vi "live view D05.vi"() -> ()   [LabVIEW 2019, in "D05.lvlib"]
uses:
  D05.lvlib
  <vilib>/userDefined/High Color/IMAQdx.ctl
  <vilib>/vision/Image Controls.llb/IMAQ Image.ctl
  <vilib>/measure/mamon.llb/Trigger Detection for 1 Channel.vi
  <vilib>/measure/NI_MAPro.lvlib
  Calibration Lib.lvlib
  database.lvlib
  <vilib>/vision/driver/NI_Vision_Acquisition_Software.lvlib
panel:
  out "error out":errorcluster
  in  "snapshot":bool
  out "projector D30 error":errorcluster
  in  "Path":path
  in  "Verify Calibration D29":bool caption="capture grab"
  out "factor":sgl
  out "transform matrix":sgl[](array[numeric])
  in  "Method 2 save D30":bool caption="capture grab"
  in  "Method 1 Save D30":bool caption="Saving txt"
  in  "Close":bool
  out "Average Result":string="Average Result"
  out ">18  A":dbl(slide)=1.0 caption=">18 mm" scale=0.0..100.0
  out "16-18  A":dbl(slide)=1.0 caption="16-18 mm" scale=0.0..100.0
  out "14-16  A":dbl(slide)=1.0 caption="14-16 mm" scale=0.0..100.0
  out "12.5-14 A":dbl(slide)=1.0 caption="12.5-14 mm" scale=0.0..100.0
  out "10-12.5  A":dbl(slide)=1.0 caption="10-12.5 mm" scale=0.0..100.0 scale format="%#_4f"
  out "8-10  A":dbl(slide)=1.0 caption="8-10 mm" scale=0.0..100.0
  out "6.3-8  A":dbl(slide)=1.0 caption="6.3-8 mm" scale=0.0..100.0
  out "<6.3  A":dbl(slide)=1.0 caption="<6.3 mm" scale=0.0..100.0
  out "Live Result":string="Live Result"
  out ">18  L":dbl(slide)=1.0 caption=">18 mm" scale=0.0..100.0
  out "Live View":T1(plugin-control) caption="Disc 26"
  out "16-18  L":dbl(slide)=1.0 caption="16-18 mm" scale=0.0..100.0
  out "14-16  L":dbl(slide)=1.0 caption="14-16 mm" scale=0.0..100.0
  out "12.5-14 L":dbl(slide)=1.0 caption="12.5-14 mm" scale=0.0..100.0
  out "10-12.5  L":dbl(slide)=1.0 caption="10-12.5 mm" scale=0.0..100.0 scale format="%#_4f"
  out "8-10  L":dbl(slide)=1.0 caption="8-10 mm" scale=0.0..100.0
  out "6.3-8  L":dbl(slide)=1.0 caption="6.3-8 mm" scale=0.0..100.0
  out "<6.3  L":dbl(slide)=1.0 caption="<6.3 mm" scale=0.0..100.0
  out "disc name":string="Live Info Disc 05"
  out "dsgs":string="DSGS"
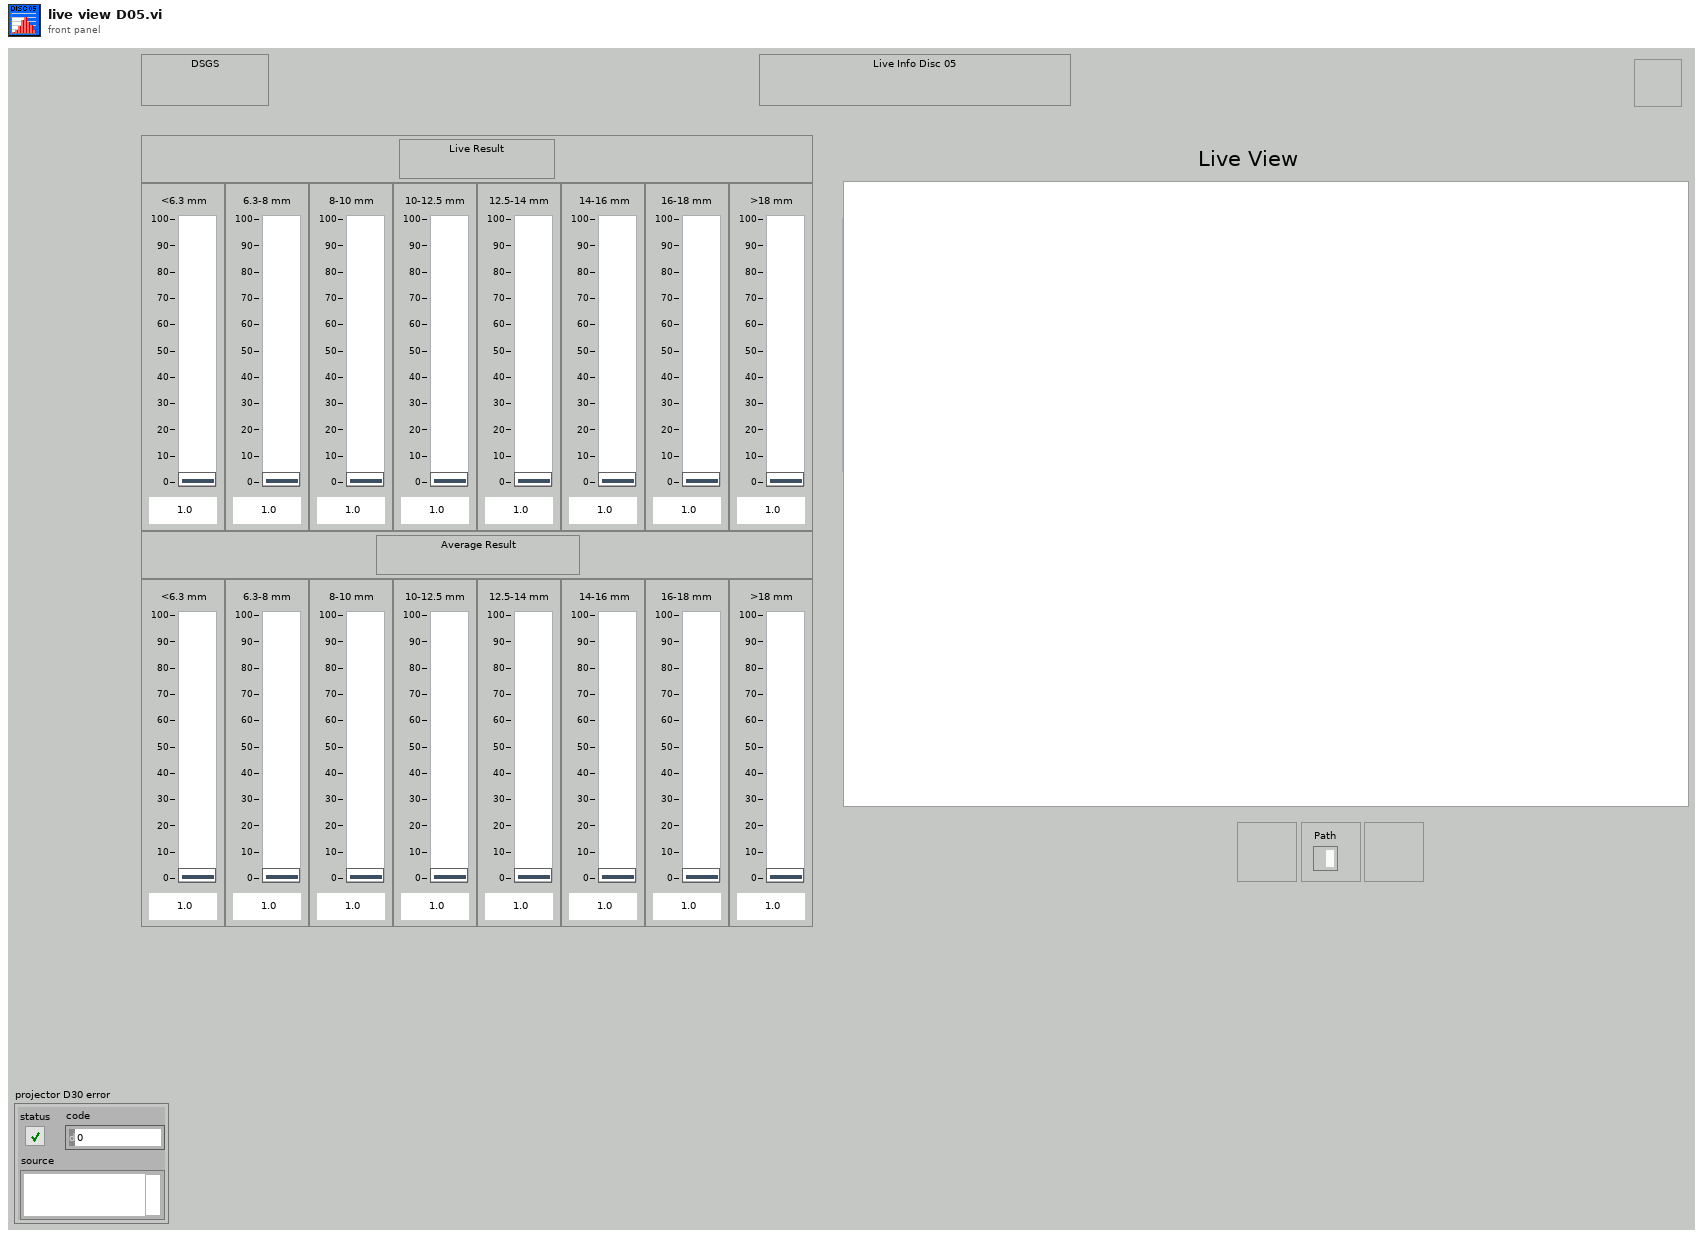
[diagram p1: front panel]
types:
  T1 = typedef "IMAQ Image.ctl" = refnum<image>
  T2 = typedef "IMAQdx.ctl" = refnum<k21>
  T3 = enum8{"Enabled", "Disabled", "Disabled and Grayed Out"}
  T4 = cluster{"date/time string":string, "date/time string":string, "date/time string":string, string, "spreadsheet string":string, string}
  T5 = cluster{"date/time string":string, "date/time string":string, string, "Value":dbl, "Value":dbl, "Value":dbl, "Value":dbl, "Value":dbl, "Value":dbl, "Value":dbl, "Value":dbl}
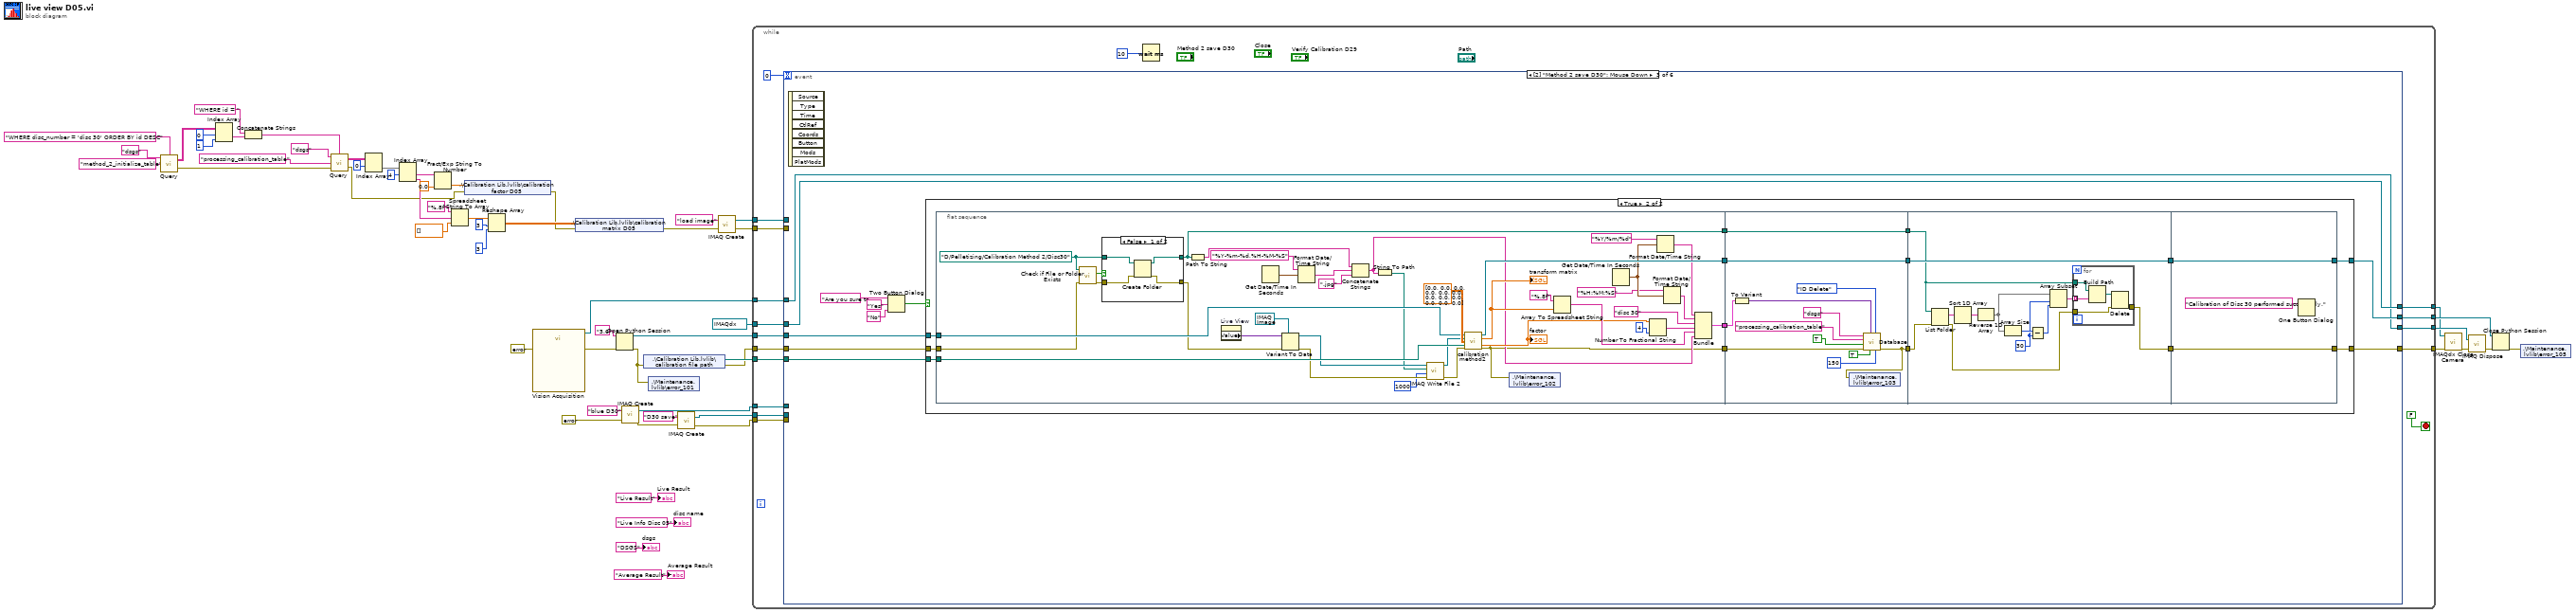
[diagram p0: block diagram]
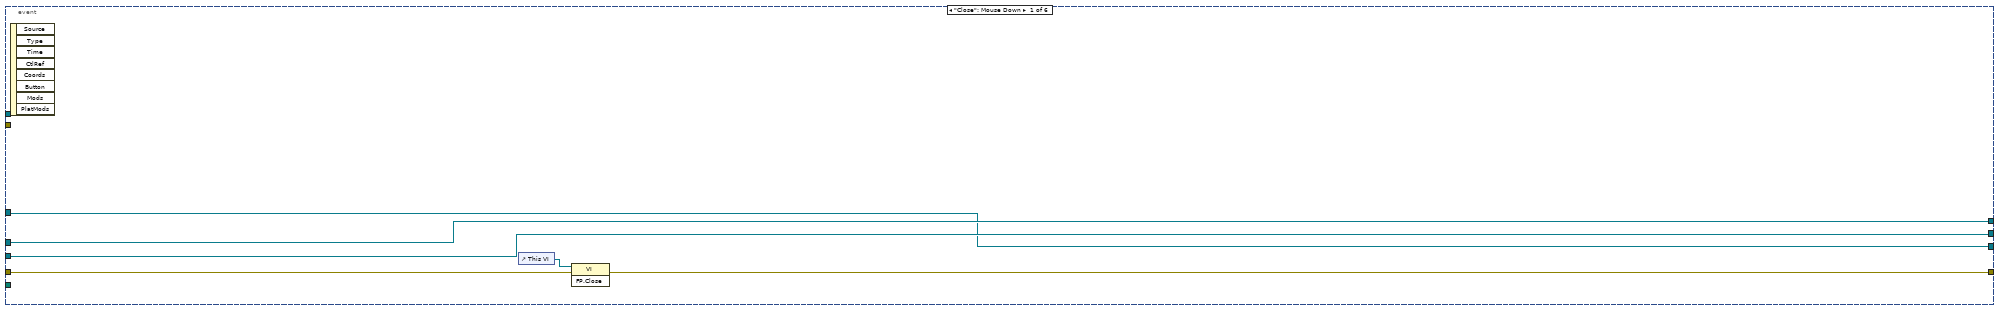
[diagram p2: hidden frame]
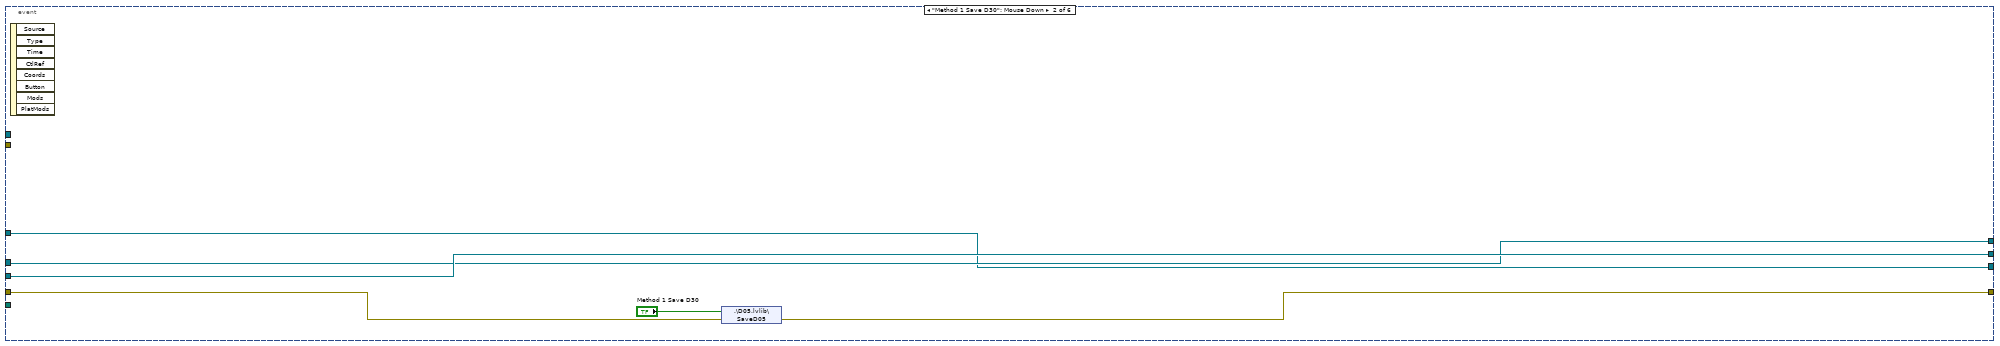
[diagram p3: hidden frame]
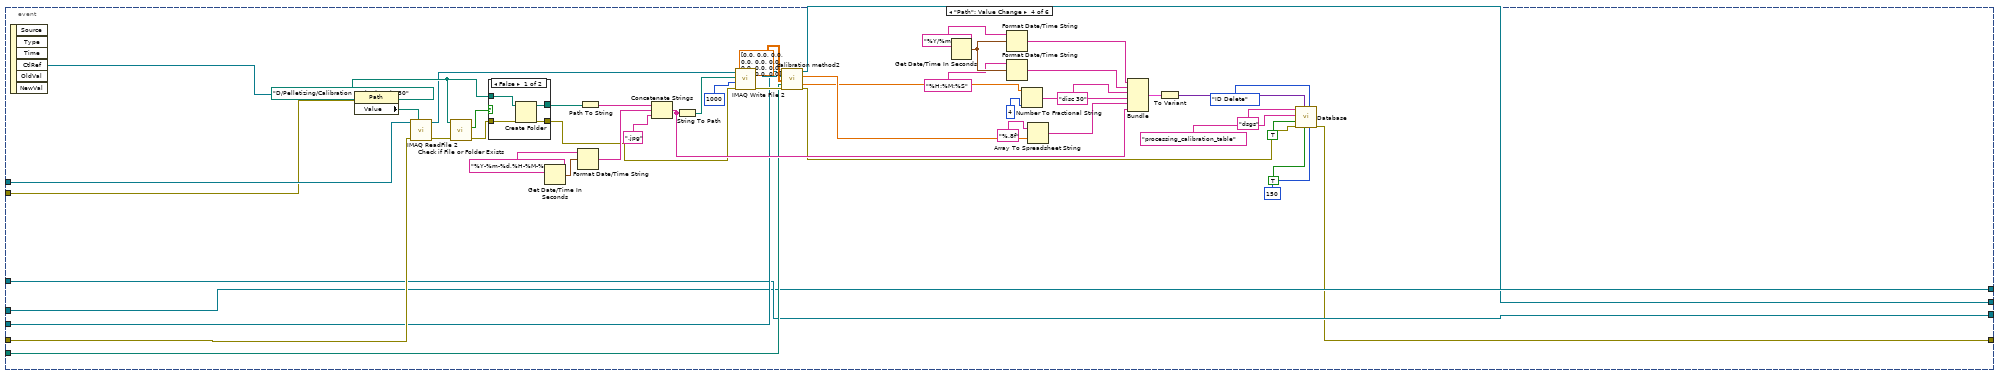
[diagram p6: hidden frame]
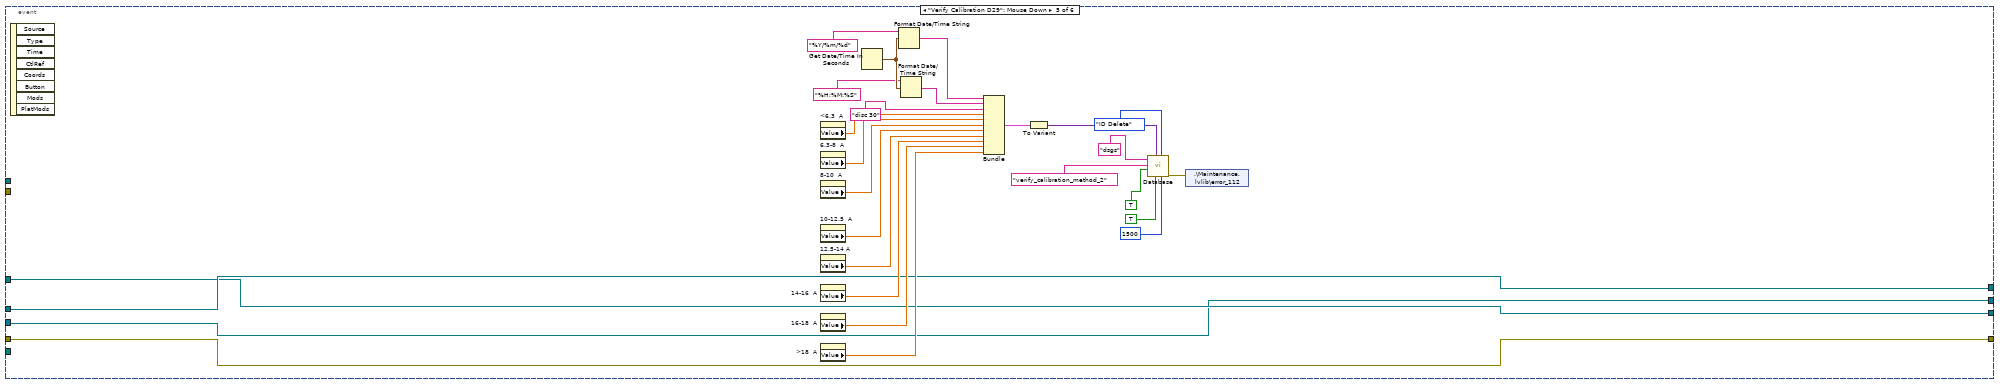
[diagram p8: hidden frame]
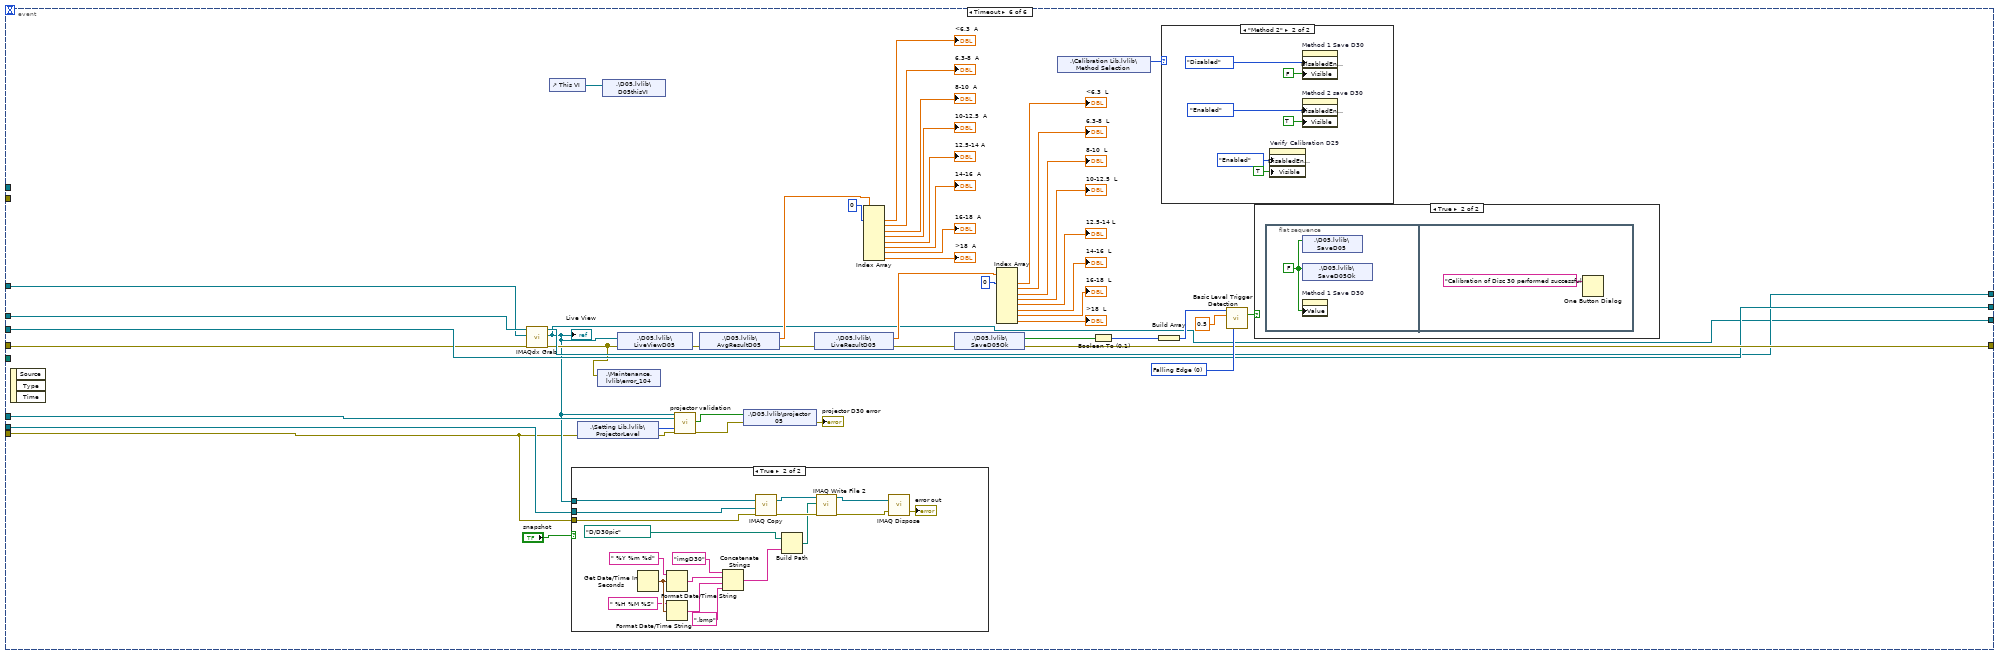
[diagram p9: hidden frame]
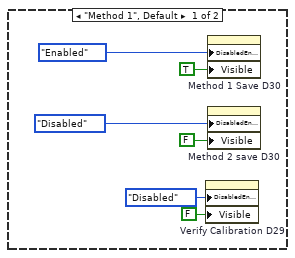
[diagram p11: hidden frame]
diagram:
  n1 = call "Query.vi"("Condition"="WHERE disc_number = 'disc 30' ORDER BY id DESC", "Table Name"="method_2_initialize_table", "Connection Name"="dsgs") -> ("Error out"=w28:errorcluster, "data"=w33:string[][])  [unwired: 1 in]
  n2 = Index Array(array=w33, index (row)=0, index (col)=1 ("disabled index (col)")) -> (element=w26:string)
  n3 = Concatenate Strings("WHERE id = " ("string"), w26) -> (w25:string)
  n4 = call "Query.vi"("Condition"=w25, "Error in"=w28, "Table Name"="processing_calibration_table", "Connection Name"="dsgs") -> ("Error out"=w9:errorcluster, "data"=w24:string[][])
  n5 = Index Array(array=w24, index (row)=0) -> (element=w22:string[])  [unwired: 1 in]
  n6 = Index Array(array=w22, index #1=4 ("index")) -> (element #1=w20:string, element #2=w12:string)  [unwired: 1 in]
  n7 = Fract/Exp String To Number(string=w20, default (0 dbl)=sgl 0.0 ("default (0 DBL)")) -> (number=w19:sgl)  [unwired: 2 in, 1 out]
  n8 = Spreadsheet String To Array(format string="%.8f", spreadsheet string=w12, array type (2D Dbl)=sgl[] []) -> (array=w16:sgl[])  [unwired: 1 in]
  n9 = shared-variable ".\\Calibration Lib.lvlib\\calibration factor D05"(w19, error in=w9) -> (error out=w10:errorcluster)
  n10 = Reshape Array(w16, 3 ("dimension size"), 3 ("dimension size")) -> (w11:sgl[][])
  n11 = call "Vision Acquisition"("error in"=errorcluster {"status"=FALSE, "code"=0, "source"=""}) -> ("Image Out"=w45:T1, "error out"=w44:errorcluster)  [unwired: 24 in, 1 out]
  n12 = shared-variable ".\\Calibration Lib.lvlib\\calibration matrix D05"(w11, error in=w10) -> (error out=w8:errorcluster)
  n13 = Open Python Session(python version="3.6" ("Python version"), 3:w44) -> (session out=w54:refnum<k35>, error out=w40:errorcluster)  [unwired: 1 in]
  n14 = call "IMAQ Create"("Image Name"="blue D30", "error in (no error)"=errorcluster {"status"=FALSE, "code"=0, "source"=""}) -> ("New Image"=w5:T1, "error out"=w4:errorcluster)  [unwired: 3 in]
  n15 = shared-variable ".\\Calibration Lib.lvlib\\calibration file path"(error in=w40) -> (w43:path, error out=w42:errorcluster)
  n16 = shared-variable ".\\Maintenance.lvlib\\error_101"(w40) -> ()  [unwired: 1 in, 1 out]
  n17 = call "IMAQ Create"("Image Name"="D30 save", "error in (no error)"=w4) -> ("New Image"=w1:T1, "error out"=w3:errorcluster)  [unwired: 3 in]
  n18 = call "IMAQ Create"("Image Name"="load image", "error in (no error)"=w8) -> ("New Image"=w39:T1, "error out"=w38:errorcluster)  [unwired: 3 in]
  n19 = while {
    tunnel: w54 -> [w74]
    tunnel: w43 -> [w73]
    tunnel: w42 -> [w72]
    tunnel: w45 -> [w70]
    tunnel: [w69] -> w53
    tunnel: [w68] -> w50
    tunnel: [w67] -> w52
    tunnel: T2 "disc30" ("Session In") -> [w66]
    tunnel: [w65] -> w47
    tunnel: w39 -> [w64]
    tunnel: w38 -> [w63]
    tunnel: w5 -> [w62]
    tunnel: w3 -> [w61]
    tunnel: w1 -> [w60]
    stop <- FALSE stop-if-true
    n20 = event shown="[2] \"Method 2 save D30\": Mouse Down" {
      selector: _ -> [_ _ _ _ _ _]
      dyn-events: _ -> [_ _ _ _ _ _]
      timeout: 0 -> [_ _ _ _ _ _]
      tunnel: w74 -> [w80 w86 w99 w196 w250 w290]
      tunnel: w73 -> [_ _ w98 w197 _ _]
      tunnel: [w82 w88 w93 w193 w253 w293] -> w68
      tunnel: w72 -> [w81 w87 w97 w198 w253 w286]
      tunnel: w70 -> [w77 w84 w94 w195 w251 w288]
      tunnel: [w77 w84 w94 w195 w251 w277] -> w69
      tunnel: [w80 w86 w96 w192 w250 w290] -> w67
      tunnel: w66 -> [w78 w85 w95 w194 w252 w289]
      tunnel: [w78 w85 w95 w194 w252 w287] -> w65
      tunnel: w64 -> [_ _ _ w200 _ _]
      tunnel: w63 -> [_ _ _ w199 _ _]
      tunnel: w62 -> [_ _ _ _ _ w279]
      tunnel: w61 -> [_ _ _ _ _ w275]
      tunnel: w60 -> [_ _ _ _ _ w276]
      event "Close": Mouse Down {
        n21 = event-data() -> ()  [unwired: 1 in, 8 out]
        n22 = control-ref of="This VI"() -> (w79:refnum<vi>)
        n23 = invoke class="VI" method="FP.Close"(reference=w79, error in=w81) -> (error out=w82:errorcluster)  [unwired: 1 in, 2 out]
      }
      event "Method 1 Save D30": Mouse Down {
        n24 = event-data() -> ()  [unwired: 1 in, 8 out]
        n25 = shared-variable ".\\D05.lvlib\\SaveD05"("Method 1 Save D30", error in=w87) -> (error out=w88:errorcluster)
      }
      event "Method 2 save D30": Mouse Down {
        n26 = event-data() -> ()  [unwired: 1 in, 8 out]
        n27 = Two Button Dialog(message="Are you sure to calibration Disc 30?", 1:"No" ("F button name (\"Cancel\")"), 2:"Yes" ("T button name (\"OK\")")) -> (T button?=w89:bool)
        n28 = case shown="True" w89 {
          tunnel: w99 -> [w100 w108]
          tunnel: w98 -> [_ w107]
          tunnel: w97 -> [w101 w106]
          tunnel: [w100 w105] -> w96
          tunnel: [w101 w104] -> w93
          frame False {
          }
          frame True {
            n29 = flat-sequence {
              tunnel: [w153] -> w115
              tunnel: [w119] -> w114
              tunnel: [w144] -> w113
              tunnel: w106 -> [w125]
              tunnel: w107 -> [w143]
              tunnel: w108 -> [w135]
              tunnel: [w118] -> w112
              tunnel: w115 -> [w171]
              tunnel: w114 -> [w169]
              tunnel: w113 -> [w164]
              tunnel: [w171] -> w111
              tunnel: [w165] -> w110
              tunnel: [w162] -> w109
              tunnel: w112 -> [w162]
              tunnel: w111 -> [w183]
              tunnel: w110 -> [w173]
              tunnel: w109 -> [w172]
              tunnel: [w183] -> w103
              tunnel: [w174] -> w102
              tunnel: [w190] -> w104
              tunnel: [w191] -> w105
              tunnel: w103 -> [w191]
              tunnel: w102 -> [w190]
              frame #0 {
                w129 = path "D:/Pelletizing/Calibration Method 2/Disc30" ("path")
                n30 = call <vilib>:"Check if File or Folder Exists.vi"("error in (no error)"=w125, "path"=w129) -> ("error out"=w127:errorcluster, "file or folder exists?"=w130:bool)  [unwired: 7 in, 1 out]
                n31 = case shown="False" w130 {
                  tunnel: [w155 w159] -> w118
                  tunnel: w129 -> [w157 w159]
                  tunnel: w127 -> [w156 w158]
                  tunnel: [w154 w158] -> w124
                  frame False {
                    n32 = Create Folder(path (use dialog)=w157, error in=w156) -> (created path=w155:path, error out=w154:errorcluster)  [unwired: 1 in, 1 out]
                  }
                  frame True {
                  }
                }
                n33 = Path To String(path=w118) -> (string=w128:string)
                n34 = property on="Live View" class="ImageControl"() -> ("Value"=w142:variant)  [unwired: 2 in, 2 out]
                n35 = Get Date/Time In Seconds() -> (seconds since 1Jan1904=w134:timestamp)
                n36 = Variant To Data(error in=w124, type=T1 refnum ("New Image"), Variant=w142) -> (data=w123:T1, error out=w122:errorcluster)
                n37 = Format Date/Time String(time format string (%c)="%Y-%m-%d,%H-%M-%S", seconds (now)=w134) -> (date/time string=w132:string)  [unwired: 1 in]
                n38 = Concatenate Strings(w128, w132, ".jpg" ("string")) -> (w126:string)
                n39 = String To Path(string=w126) -> (path=w121:path)
                n40 = call-poly "IMAQ Write File 2"("error in (no error)"=w122, "Image Quality"=u32 1000, "File Path"=w121, "Image"=w123) -> ("error out"=w116:errorcluster, "Image Out (duplicate)"=w117:T1)  [unwired: 6 in]
                n41 = call "calibration method2.vi"("session in"=w135, "Image IN"=w117, "initialize matrix"=sgl[][] [[0.0, 0.0, 0.0], [0.0, 0.0, 0.0], [0.0, 0.0, 0.0], [0.0, 0.0, 0.0]] ("(4*3) array"), "module path"=w143, "error in"=w116) -> ("session out"=w153:refnum<k35>, "calibration vector"=w137:sgl[], "factor"=w139:sgl, "error out"=w119:errorcluster)  [unwired: 6 in, 1 out]
                "factor" <- w139
                "transform matrix" <- w137
                n42 = shared-variable ".\\Maintenance.lvlib\\error_102"(w119) -> ()  [unwired: 1 in, 1 out]
                n43 = Array To Spreadsheet String(array=w137, 3:"%.8f" ("format string")) -> (spreadsheet string=w145:string)  [unwired: 1 in]
                n44 = Get Date/Time In Seconds() -> (seconds since 1Jan1904=w150:timestamp)
                n45 = Number To Fractional String(number=w139, precision (6)=i16 4) -> (F-format string=w146:string)  [unwired: 2 in]
                n46 = Format Date/Time String(time format string (%c)="%Y/%m/%d", seconds (now)=w150) -> (date/time string=w151:string)  [unwired: 1 in]
                n47 = Format Date/Time String(time format string (%c)="%H:%M:%S", seconds (now)=w150) -> (date/time string=w152:string)  [unwired: 1 in]
                n48 = Bundle("date/time string"=w151, "date/time string"=w152, "date/time string"="disc 30", w146, "spreadsheet string"=w145, w126) -> (w144:T4)  [unwired: 1 in]
              }
              frame #1 {
                n49 = To Variant(anything=w164) -> (Variant=w163:variant)
                n50 = call "Database.vi"("Maximum Row"=150, "Enum"=enum16{"ID Delete", "Time Delete"}."ID Delete", "Delete row?"=TRUE, "Data"=w163, "Error in"=w169, "Auto Increment ID?"=TRUE, "Table"="processing_calibration_table", "Connection"="dsgs") -> ("Error out"=w165:errorcluster)  [unwired: 3 in]
                n51 = shared-variable ".\\Maintenance.lvlib\\error_103"(w165) -> ()  [unwired: 1 in, 1 out]
              }
              frame #2 {
                w176 = 30 ("index")
                n52 = List Folder(path=w172, error in=w173) -> (filenames=w177:string[], error out=w175:errorcluster)  [unwired: 2 in, 2 out]
                n53 = Sort 1D Array(array=w177) -> (sorted array=w178:string[])
                n54 = Reverse 1D Array(array=w178) -> (reversed array=w179:string[])
                n55 = Array Size(array=w179) -> (size(s)=w180:i32)
                n56 = Subtract(x=w180, y=w176) -> (x-y=w181:i32)
                n57 = Array Subset(array=w179, index=w176, length=w181) -> (w182:string[])
                n58 = for {
                  tunnel: w182 -> [w187] mode=indexing
                  tunnel: w172 -> [w188]
                  tunnel: [w185] -> w174
                  tunnel: w175 -> [w184]
                  n59 = Build Path(base path=w188, name or relative path=w187) -> (appended path=w186:path)
                  n60 = Delete(path (use dialog)=w186, error in=w184) -> (error out=w185:errorcluster)  [unwired: 3 in, 2 out]
                }
              }
              frame #3 {
                n61 = One Button Dialog(message="Calibration of Disc 30 performed successfully.") -> ()  [unwired: 1 in, 1 out]
              }
            }
          }
        }
      }
      event "Path": Value Change {
        w233 = path "D:/Pelletizing/Calibration Method 2/Disc30" ("path")
        n62 = event-data() -> ("CtlRef"=w201:refnum<vi>)  [unwired: 1 in, 5 out]
        n63 = property class="Path"(reference=w201, error in=w199) -> ("Value"=w228:path)  [unwired: 2 out]
        n64 = call "IMAQ ReadFile 2"("File Path"=w228, "error in (no error)"=w198, "Image"=w200) -> ("error out"=w226:errorcluster, "Image Out"=w227:T1)  [unwired: 4 in, 3 out]
        n65 = call <vilib>:"Check if File or Folder Exists.vi"("error in (no error)"=w226, "path"=w233) -> ("error out"=w230:errorcluster, "file or folder exists?"=w234:bool)  [unwired: 7 in, 1 out]
        n66 = case shown="False" w234 {
          tunnel: [w243 w247] -> w232
          tunnel: w233 -> [w245 w247]
          tunnel: w230 -> [w244 w246]
          tunnel: [w242 w246] -> w203
          frame False {
            n67 = Create Folder(path (use dialog)=w245, error in=w244) -> (created path=w243:path, error out=w242:errorcluster)  [unwired: 1 in, 1 out]
          }
          frame True {
          }
        }
        n68 = Get Date/Time In Seconds() -> (seconds since 1Jan1904=w238:timestamp)
        n69 = Format Date/Time String(time format string (%c)="%Y-%m-%d,%H-%M-%S", seconds (now)=w238) -> (date/time string=w236:string)  [unwired: 1 in]
        n70 = Path To String(path=w232) -> (string=w231:string)
        n71 = Concatenate Strings(w231, w236, ".jpg" ("string")) -> (w214:string)
        n72 = String To Path(string=w214) -> (path=w229:path)
        n73 = call-poly "IMAQ Write File 2"("error in (no error)"=w203, "Image Quality"=u32 1000, "File Path"=w229, "Image"=w227) -> ("error out"=w240:errorcluster, "Image Out (duplicate)"=w225:T1)  [unwired: 6 in]
        n74 = call "calibration method2.vi"("session in"=w196, "Image IN"=w225, "initialize matrix"=sgl[][] [[0.0, 0.0, 0.0], [0.0, 0.0, 0.0], [0.0, 0.0, 0.0], [0.0, 0.0, 0.0]] ("(4*3) array"), "module path"=w197, "error in"=w240) -> ("session out"=w192:refnum<k35>, "calibration vector"=w213:sgl[], "factor"=w212:sgl, "error out"=w202:errorcluster)  [unwired: 6 in, 1 out]
        n75 = Get Date/Time In Seconds() -> (seconds since 1Jan1904=w222:timestamp)
        n76 = Format Date/Time String(time format string (%c)="%Y/%m/%d", seconds (now)=w222) -> (date/time string=w223:string)  [unwired: 1 in]
        n77 = Format Date/Time String(time format string (%c)="%H:%M:%S", seconds (now)=w222) -> (date/time string=w224:string)  [unwired: 1 in]
        n78 = Number To Fractional String(number=w212, precision (6)=i16 4) -> (F-format string=w218:string)  [unwired: 2 in]
        n79 = Array To Spreadsheet String(array=w213, 3:"%.8f" ("format string")) -> (spreadsheet string=w217:string)  [unwired: 1 in]
        n80 = Bundle("date/time string"=w223, "date/time string"=w224, "date/time string"="disc 30", w218, "spreadsheet string"=w217, w214) -> (w204:T4)  [unwired: 1 in]
        n81 = To Variant(anything=w204) -> (Variant=w207:variant)
        n82 = call "Database.vi"("Maximum Row"=150, "Enum"=enum16{"ID Delete", "Time Delete"}."ID Delete", "Delete row?"=TRUE, "Data"=w207, "Error in"=w202, "Auto Increment ID?"=TRUE, "Table"="processing_calibration_table", "Connection"="dsgs") -> ("Error out"=w193:errorcluster)  [unwired: 3 in]
      }
      event "Verify Calibration D29": Mouse Down {
        n83 = event-data() -> ()  [unwired: 1 in, 8 out]
        n84 = property on="<6.3  A" class="Slide (strict)"() -> ("Value"=w271:dbl)  [unwired: 2 in, 2 out]
        n85 = property on="6.3-8  A" class="Slide (strict)"() -> ("Value"=w270:dbl)  [unwired: 2 in, 2 out]
        n86 = property on="8-10  A" class="Slide (strict)"() -> ("Value"=w269:dbl)  [unwired: 2 in, 2 out]
        n87 = property on="10-12.5  A" class="Slide (strict)"() -> ("Value"=w268:dbl)  [unwired: 2 in, 2 out]
        n88 = property on="12.5-14 A" class="Slide (strict)"() -> ("Value"=w267:dbl)  [unwired: 2 in, 2 out]
        n89 = property on="14-16  A" class="Slide (strict)"() -> ("Value"=w266:dbl)  [unwired: 2 in, 2 out]
        n90 = property on="16-18  A" class="Slide (strict)"() -> ("Value"=w265:dbl)  [unwired: 2 in, 2 out]
        n91 = property on=">18  A" class="Slide (strict)"() -> ("Value"=w264:dbl)  [unwired: 2 in, 2 out]
        n92 = Get Date/Time In Seconds() -> (seconds since 1Jan1904=w274:timestamp)
        n93 = Format Date/Time String(time format string (%c)="%Y/%m/%d", seconds (now)=w274) -> (date/time string=w273:string)  [unwired: 1 in]
        n94 = Format Date/Time String(time format string (%c)="%H:%M:%S", seconds (now)=w274) -> (date/time string=w272:string)  [unwired: 1 in]
        n95 = Bundle("date/time string"=w273, "date/time string"=w272, "disc 30", "Value"=w271, "Value"=w270, "Value"=w269, "Value"=w268, "Value"=w267, "Value"=w266, "Value"=w265, "Value"=w264) -> (w263:T5)  [unwired: 1 in]
        n96 = To Variant(anything=w263) -> (Variant=w262:variant)
        n97 = call "Database.vi"("Maximum Row"=1500, "Enum"=enum16{"ID Delete", "Time Delete"}."ID Delete", "Delete row?"=TRUE, "Data"=w262, "Auto Increment ID?"=TRUE, "Table"="verify_calibration_method_2", "Connection"="dsgs") -> ("Error out"=w261:errorcluster)  [unwired: 4 in]
        n98 = shared-variable ".\\Maintenance.lvlib\\error_112"(w261) -> ()  [unwired: 1 in, 1 out]
      }
      event Timeout {
        w298 = u16 0 items=["Falling Edge", "Rising Edge"] ("trigger slope")
        n99 = event-data() -> ()  [unwired: 1 in, 3 out]
        n100 = call <vilib>:"IMAQdx Grab.vi"("error in"=w286, "Image In"=w288, "Session In"=w289) -> ("error out"=w285:errorcluster, "Image Out"=w277:T1, "Session Out"=w287:T2)  [unwired: 1 in, 5 out]
        "Live View" <- w277
        n101 = control-ref of="This VI"() -> (w291:refnum<vi>)
        n102 = case shown="True" "snapshot" {
          tunnel: w276 -> [_ w340]
          tunnel: w277 -> [_ w339]
          tunnel: w275 -> [_ w323]
          frame False {
          }
          frame True {
            n103 = Get Date/Time In Seconds() -> (seconds since 1Jan1904=w333:timestamp)
            n104 = Format Date/Time String(time format string (%c)=" %Y %m %d", seconds (now)=w333) -> (date/time string=w329:string)  [unwired: 1 in]
            n105 = Format Date/Time String(time format string (%c)=" %H %M %S", seconds (now)=w333) -> (date/time string=w328:string)  [unwired: 1 in]
            n106 = Concatenate Strings("imgD30" ("string"), w329, w328, ".bmp" ("string")) -> (w326:string)
            n107 = call "IMAQ Copy"("error in (no error)"=w323, "Image Dst"=w340, "Image Src"=w339) -> ("error out"=w337:errorcluster, "Image Dst Out"=w338:T1)  [unwired: 3 in]
            n108 = Build Path(base path=path "D:/D30pic" ("File Path"), name or relative path=w326) -> (appended path=w325:path)
            n109 = call-poly "IMAQ Write File 2"("error in (no error)"=w337, "File Path"=w325, "Image"=w338) -> ("error out"=w335:errorcluster, "Image Out (duplicate)"=w336:T1)  [unwired: 7 in]
            n110 = call "IMAQ Dispose"("Image"=w336, "error in (no error)"=w335) -> ("error out"=→"error out":errorcluster)  [unwired: 4 in]
          }
        }
        n111 = shared-variable ".\\Setting Lib.lvlib\\ProjectorLevel"(error in=w275) -> (w284:i32, error out=w283:errorcluster)
        n112 = shared-variable ".\\Maintenance.lvlib\\error_104"(w285) -> ()  [unwired: 1 in, 1 out]
        n113 = shared-variable ".\\D05.lvlib\\D05thisVI"(w291) -> ()  [unwired: 1 in, 1 out]
        n114 = shared-variable ".\\D05.lvlib\\LiveViewD05"(w277, error in=w285) -> (error out=w292:errorcluster)
        n115 = call "projector validation.vi"("Image Src"=w277, "blue channel"=w279, "on/off level"=w284, "error in (no error)"=w283) -> ("on/off"=w282:bool, "error out"=w281:errorcluster)  [unwired: 14 in]
        n116 = shared-variable ".\\D05.lvlib\\AvgResultD05"(error in=w292) -> (w313:dbl[], error out=w295:errorcluster)
        n117 = shared-variable ".\\D05.lvlib\\projector 05"(w282, error in=w281) -> (error out=→"projector D30 error":errorcluster)
        n118 = shared-variable ".\\D05.lvlib\\LiveResultD05"(error in=w295) -> (w312:dbl[], error out=w294:errorcluster)
        n119 = Index Array(array=w313, index #1=0 ("index")) -> (element #1=→"<6.3  A":dbl, element #2=→"6.3-8  A":dbl, element #3=→"8-10  A":dbl, element #4=→"10-12.5  A":dbl, element #5=→"12.5-14 A":dbl, element #6=→"14-16  A":dbl, element #7=→"16-18  A":dbl, element #8=→">18  A":dbl)  [unwired: 7 in]
        n120 = shared-variable ".\\D05.lvlib\\SaveD05Ok"(error in=w294) -> (w299:bool, error out=w293:errorcluster)
        n121 = Index Array(array=w312, index #1=0 ("index")) -> (element #1=→"<6.3  L":dbl, element #2=→"6.3-8  L":dbl, element #3=→"8-10  L":dbl, element #4=→"10-12.5  L":dbl, element #5=→"12.5-14 L":dbl, element #6=→"14-16  L":dbl, element #7=→"16-18  L":dbl, element #8=→">18  L":dbl)  [unwired: 7 in]
        n122 = shared-variable ".\\Calibration Lib.lvlib\\Method Selection"() -> (w296:enum32{"Method 1", "Method 2"})  [unwired: 1 in, 1 out]
        n123 = Boolean To (0,1)(Boolean=w299) -> (0, 1=w302:i16)
        n124 = Build Array(w302) -> (w301:i16[])
        n125 = case shown="\"Method 2\"" w296 {
          frame "Method 1", Default {
            n126 = property on="Verify Calibration D29" class="Bool (strict)"("DisabledEnum"=T3."Disabled" ("Disabled"), "Visible"=FALSE) -> ()  [unwired: 2 in, 2 out]
            n127 = property on="Method 1 Save D30" class="Bool (strict)"("DisabledEnum"=T3."Enabled" ("Disabled"), "Visible"=TRUE) -> ()  [unwired: 2 in, 2 out]
            n128 = property on="Method 2 save D30" class="Bool (strict)"("DisabledEnum"=T3."Disabled" ("Disabled"), "Visible"=FALSE) -> ()  [unwired: 2 in, 2 out]
          }
          frame "Method 2" {
            n129 = property on="Verify Calibration D29" class="Bool (strict)"("DisabledEnum"=T3."Enabled" ("Disabled"), "Visible"=TRUE) -> ()  [unwired: 2 in, 2 out]
            n130 = property on="Method 1 Save D30" class="Bool (strict)"("DisabledEnum"=T3."Disabled" ("Disabled"), "Visible"=FALSE) -> ()  [unwired: 2 in, 2 out]
            n131 = property on="Method 2 save D30" class="Bool (strict)"("DisabledEnum"=T3."Enabled" ("Disabled"), "Visible"=TRUE) -> ()  [unwired: 2 in, 2 out]
          }
        }
        n132 = call-poly <vilib>:"Basic Level Trigger Detection.vi"("signal in"=w301, "level"=0.5, "trigger slope"=w298) -> ("trigger detected?"=w297:bool)  [unwired: 10 in, 2 out]
        n133 = case shown="True" w297 {
          frame False {
          }
          frame True {
            n134 = flat-sequence {
              frame #0 {
                w353 = FALSE
                n135 = shared-variable ".\\D05.lvlib\\SaveD05Ok"(w353) -> ()  [unwired: 1 in, 1 out]
                n136 = property on="Method 1 Save D30" class="Bool (strict)"("Value"=w353) -> ()  [unwired: 2 in, 2 out]
                n137 = shared-variable ".\\D05.lvlib\\SaveD05"(w353) -> ()  [unwired: 1 in, 1 out]
              }
              frame #1 {
                n138 = One Button Dialog(message="Calibration of Disc 30 performed successfully.") -> ()  [unwired: 1 in, 1 out]
              }
            }
          }
        }
      }
    }
    n139 = Wait (ms)(milliseconds to wait=u32 10) -> ()  [unwired: 1 out]
  }
  n140 = call <vilib>:"IMAQdx Close Camera.vi"("error in"=w50, "Session In"=w47) -> ("error out"=w49:errorcluster)  [unwired: 9 in]
  n141 = call "IMAQ Dispose"("Image"=w53, "error in (no error)"=w49) -> ("error out"=w51:errorcluster)  [unwired: 4 in]
  n142 = Close Python Session(session in=w52, error in=w51) -> (11:w41:errorcluster)
  n143 = shared-variable ".\\Maintenance.lvlib\\error_105"(w41) -> ()  [unwired: 1 in, 1 out]
  "Live Result" <- "Live Result" ("Live Result")
  "Average Result" <- "Average Result" ("Average Result")
  "disc name" <- "Live Info Disc 05" ("Live Result")
  "dsgs" <- "DSGS" ("Live Result")
